vi "Report_Header.vi"(2 "Error In":errorcluster) -> (0 "Error Out":errorcluster)   [LabVIEW 2019]
uses:
  Global Variables/Global_Variables.vi
  <vilib>/Utility/file.llb/Write Delimited Spreadsheet (string).vi
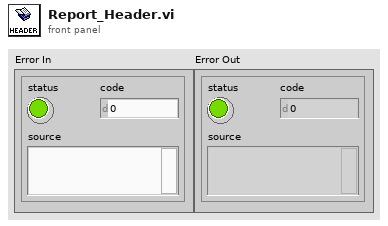
[diagram p1: front panel]
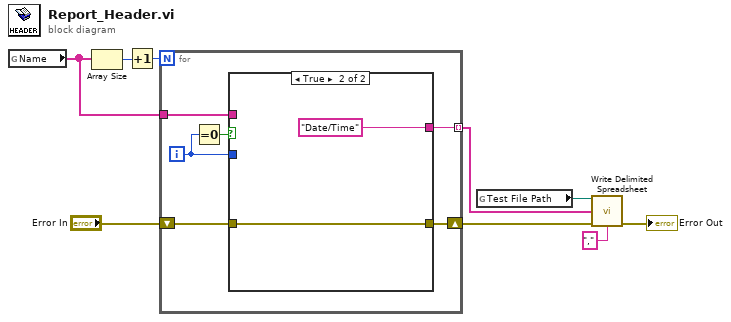
[diagram p0: block diagram]
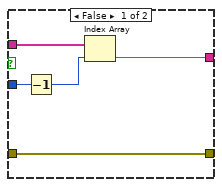
[diagram p2: hidden frame]
diagram:
  n1 = global read "Global_Variables.vi" "Name"() -> (w6:string[])
  n2 = Array Size(array=w6) -> (size(s)=w8:i32)
  n3 = Increment(x=w8) -> (x+1=w7:i32)
  n4 = for {
    N: w7 -> [_]
    shift-right: [w11] -> w5
    shift-left: "Error In" -> [w12]
    tunnel: w6 -> [w13]
    tunnel: [w10] -> w4 mode=indexing
    i -> [w14]
    n5 = Equal To 0?(x=w14) -> (x = 0?=w15:bool)
    n6 = case shown="True" w15 {
      tunnel: w14 -> [w19 _]
      tunnel: w13 -> [w18 _]
      tunnel: w12 -> [w20 w22]
      tunnel: [w20 w22] -> w11
      tunnel: [w16 "Date/Time"] -> w10
      frame False {
        n7 = Decrement(x=w19) -> (x-1=w17:i32)
        n8 = Index Array(array=w18, index=w17) -> (element=w16:string)
      }
      frame True {
      }
    }
  }
  n9 = global read "Global_Variables.vi" "Test File Path"() -> (w2:path)
  n10 = call-poly <vilib>:"Write Delimited Spreadsheet.vi"("file path (dialog if empty)"=w2, "1D data"=w4, "error in (no error)"=w5, "delimiter (\\t)"="," ("delimiter (\\t)")) -> ("error out"=→"Error Out":errorcluster)  [unwired: 10 in, 1 out]
